vi "GaussianProcessRegressor.vi"(8 "error in":errorcluster) -> (0 "error out":errorcluster, 3 "out":refnum<class "GaussianProcessRegressor.lvclass">)   [LabVIEW 2020]
doc: "Gaussian process regression (GPR).\n\n The implementation is based on Algorithm 2.1 of Gaussian Processes\n for Machine Learning (GPML) by Rasmussen and Williams.\n\n In addition to standard scikit-learn estimator API,\n GaussianProcessRegressor:\n\n * allows prediction without prior fitting (based on the GP prior)\n * provides an additional method sample_y(X), which evaluates samples\n drawn from the GPR (prior or posterior) at given inputs\n * exposes a method log_marginal_likelihood(theta), which can be used\n externally for other ways of selecting hyperparameters, e.g., via\n Markov chain Monte Carlo.\n\n Read more in the :ref:`User Guide <gaussian_process>`.\n\n .. versionadded:: 0.18\n\n Parameters\n ----------\n kernel : kernel instance, default=None\n The kernel specifying the covariance function of the GP. If None is\n passed, the kernel ``ConstantKernel(1.0, constant_value_bounds=\"fixed\"\n * RBF(1.0, length_scale_bounds=\"fixed\")`` is used as default. Note that\n the kernel hyperparameters are optimized during fitting unless the\n bounds are marked as \"fixed\".\n\n alpha : float or ndarray of shape (n_samples,), default=1e-10\n Value added to the diagonal of the kernel matrix during fitting.\n This can prevent a potential numerical issue during fitting, by\n ensuring that the calculated values form a positive definite matrix.\n It can also be interpreted as the variance of additional Gaussian\n measurement noise on the training observations. Note that this is\n different from using a `WhiteKernel`. If an array is passed, it must\n have the same number of entries as the data used for fitting and is\n used as datapoint-dependent noise level. Allowing to specify the\n noise level directly as a parameter is mainly for convenience and\n for consistency with Ridge.\n\n optimizer : \"fmin_l_bfgs_b\" or callable, default=\"fmin_l_bfgs_b\"\n Can either be one of the internally supported optimizers for optimizing\n the kernel's parameters, specified by a string, or an externally\n defined optimizer passed as a callable. If a callable is passed, it\n must have the signature::\n\n def optimizer(obj_func, initial_theta, bounds):\n # * 'obj_func' is the objective function to be minimized, which\n # takes the hyperparameters theta as parameter and an\n # optional flag eval_gradient, which determines if the\n # gradient is returned additionally to the function value\n # * 'initial_theta': the initial value for theta, which can be\n # used by local optimizers\n # * 'bounds': the bounds on the values of theta\n ....\n # Returned are the best found hyperparameters theta and\n # the corresponding value of the target function.\n return theta_opt, func_min\n\n Per default, the 'L-BGFS-B' algorithm from scipy.optimize.minimize\n is used. If None is passed, the kernel's parameters are kept fixed.\n Available internal optimizers are::\n\n 'fmin_l_bfgs_b'\n\n n_restarts_optimizer : int, default=0\n The number of restarts of the optimizer for finding the kernel's\n parameters which maximize the log-marginal likelihood. The first run\n of the optimizer is performed from the kernel's initial parameters,\n the remaining ones (if any) from thetas sampled log-uniform randomly\n from the space of allowed theta-values. If greater than 0, all bounds\n must be finite. Note that n_restarts_optimizer == 0 implies that one\n run is performed.\n\n normalize_y : bool, default=False\n Whether the target values y are normalized, the mean and variance of\n the target values are set equal to 0 and 1 respectively. This is\n recommended for cases where zero-mean, unit-variance priors are used.\n Note that, in this implementation, the normalisation is reversed\n before the GP predictions are reported.\n\n .. versionchanged:: 0.23\n\n copy_X_train : bool, default=True\n If True, a persistent copy of the training data is stored in the\n object. Otherwise, just a reference to the training data is stored,\n which might cause predictions to change if the data is modified\n externally.\n\n random_state : int, RandomState instance or None, default=None\n Determines random number generation used to initialize the centers.\n Pass an int for reproducible results across multiple function calls.\n See :term: `Glossary <random_state>`.\n\n Attributes\n ----------\n X_train_ : array-like of shape (n_samples, n_features) or list of object\n Feature vectors or other representations of training data (also\n required for prediction).\n\n y_train_ : array-like of shape (n_samples,) or (n_samples, n_targets)\n Target values in training data (also required for prediction)\n\n kernel_ : kernel instance\n The kernel used for prediction. The structure of the kernel is the\n same as the one passed as parameter but with optimized hyperparameters\n\n L_ : array-like of shape (n_samples, n_samples)\n Lower-triangular Cholesky decomposition of the kernel in ``X_train_``\n\n alpha_ : array-like of shape (n_samples,)\n Dual coefficients of training data points in kernel space\n\n log_marginal_likelihood_value_ : float\n The log-marginal-likelihood of ``self.kernel_.theta``\n\n \nAvailable methods:\nGet Attributes\nGet Params\nSet Params"
uses:
  Gaussian_process/GaussianProcessRegressor/GaussianProcessRegressor.lvclass
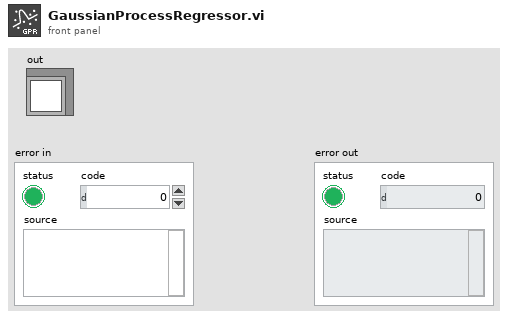
[diagram p1: front panel]
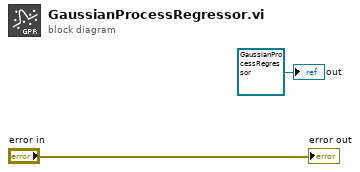
[diagram p0: block diagram]
diagram:
  "out" <- refnum<class "GaussianProcessRegressor.lvclass"> refnum ("model")
  "error out" <- "error in"
